vi "Mass copy POS CONT, OUTcar.vi"() -> ()   [LabVIEW 2010]
panel:
  out "offset past match 2":i32
  out "Array":path[](array[path])
  out "All Files in Dir":path[](array[path])
  in  "Target":path
  in  "Primary":path
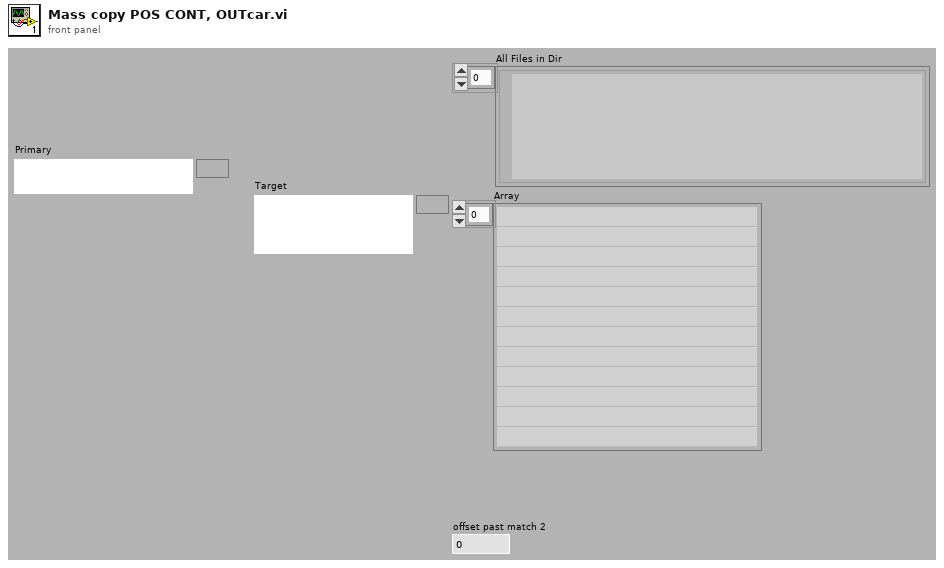
[diagram p1: front panel]
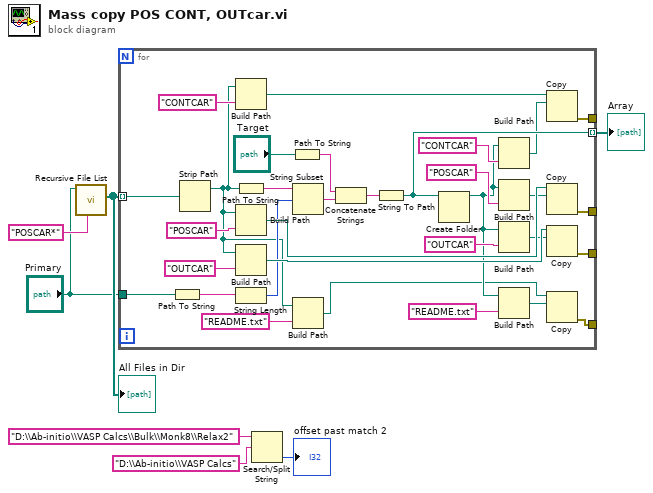
[diagram p0: block diagram]
diagram:
  n1 = call <vilib>:"Recursive File List.vi"("pattern"="POSCAR*", "Folder Path"="Primary") -> ("All Files in Dir"=w6:path[])  [unwired: 5 in, 4 out]
  "All Files in Dir" <- w6
  n2 = for {
    tunnel: w6 -> [w39] mode=indexing
    tunnel: "Primary" -> [w32]
    tunnel: [w24] -> w4 mode=indexing
    tunnel: [w11] -> _
    tunnel: [w10] -> _
    tunnel: [w9] -> _
    tunnel: [w8] -> _
    n3 = Path To String(path=w32) -> (string=w30:string)
    n4 = Strip Path(path=w39) -> (stripped path=w13:path)  [unwired: 1 out]
    n5 = Build Path(base path=w13, name or relative path="CONTCAR") -> (appended path=w33:path)
    n6 = Path To String(path=w13) -> (string=w28:string)
    n7 = Build Path(base path=w13, name or relative path="POSCAR") -> (appended path=w35:path)
    n8 = Build Path(base path=w13, name or relative path="OUTCAR") -> (appended path=w34:path)
    n9 = String Length(string=w30) -> (length=w29:i32)
    n10 = Path To String(path="Target") -> (string=w25:string)
    n11 = String Subset(string=w28, offset (0)=w29) -> (substring=w27:string)  [unwired: 1 in]
    n12 = Build Path(base path=w13, name or relative path="README.txt") -> (appended path=w12:path)
    n13 = Concatenate Strings(w25, w27) -> (w31:string)
    n14 = String To Path(string=w31) -> (path=w24:path)
    n15 = Create Folder(path (use dialog)=w24) -> (created path=w15:path)  [unwired: 2 in, 2 out]
    n16 = Build Path(base path=w15, name or relative path="CONTCAR") -> (appended path=w20:path)
    n17 = Build Path(base path=w15, name or relative path="POSCAR") -> (appended path=w19:path)
    n18 = Build Path(base path=w15, name or relative path="OUTCAR") -> (appended path=w18:path)
    n19 = Build Path(base path=w15, name or relative path="README.txt") -> (appended path=w17:path)
    n20 = Copy(10:w20, 11:w33) -> (0:w8:errorcluster)  [unwired: 3 in, 2 out]
    n21 = Copy(10:w19, 11:w35) -> (0:w9:errorcluster)  [unwired: 3 in, 2 out]
    n22 = Copy(10:w18, 11:w34) -> (0:w10:errorcluster)  [unwired: 3 in, 2 out]
    n23 = Copy(10:w17, 11:w12) -> (0:w11:errorcluster)  [unwired: 3 in, 2 out]
  }
  "Array" <- w4
  n24 = Search/Split String(string="D:\\Ab-initio\\VASP Calcs\\Bulk\\Monk8\\Relax2" ("string 2"), search string/char (-)="D:\\Ab-initio\\VASP Calcs" ("regular expression 2")) -> (offset of match=→"offset past match 2":i32)  [unwired: 1 in, 2 out]
